vi "vis_acq_disassemble_finitePostproc.vi"(7 "error in":errorcluster) -> (20 "All Images Out":T1[](array[plugin-control]), 27 "error out":errorcluster)   [LabVIEW 2013]
doc: "Creates, and edits acquisitions using the NI Vision Acquisition Express VI.\n\nThe NI Vision Acquisition Wizard is launched by placing the Express VI on the block diagram. Select an acquisition source and configure an acquisition using NI-IMAQ, NI-IMAQdx, or simulate an acquisition by reading an AVI or image files from a folder. After an acquisition is configured, select controls and indicators to be able to programmatically set in LabVIEW. Double-click the Vision Acquisition Express VI to edit the acquisition.\n\nNote: Any images created by the Express VI need to be disposed after use. Use the IMAQ Dispose.vi to cleanup the images output by the Express VI when they are no longer needed."
uses:
  <vilib>/vision/driver/Vision Acquisition Express Utility VIs.llb/Vision Acquisition Path Convert (String).vi
  <vilib>/vision/driver/NI_Vision_Acquisition_Software.lvlib
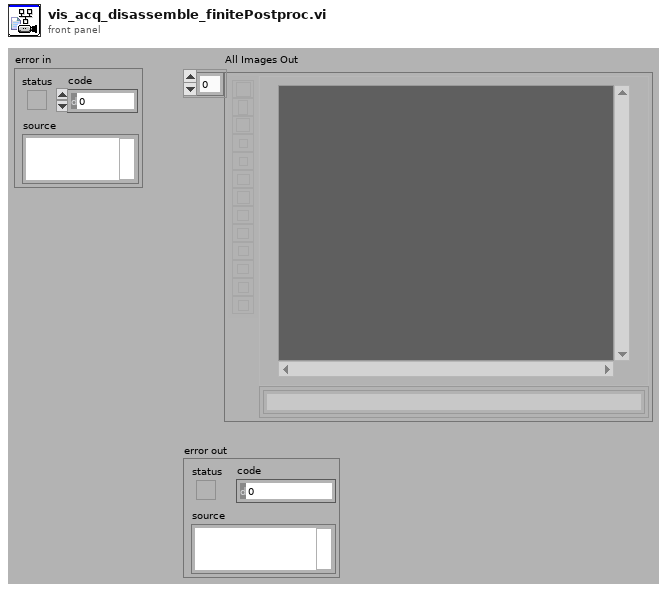
[diagram p1: front panel]
types:
  T1 = typedef "IMAQ Image.ctl" = refnum<image>
  T2 = typedef "IMAQdx.ctl" = refnum<k21>
  T3 = cluster{"File Type":string, "Quality":u32, "Compress":bool, "Lossless":bool, "Ratio":sgl, "Codec":string, "Frame Rate":u32, "Limit Frames":bool, "Max Frames":u32}
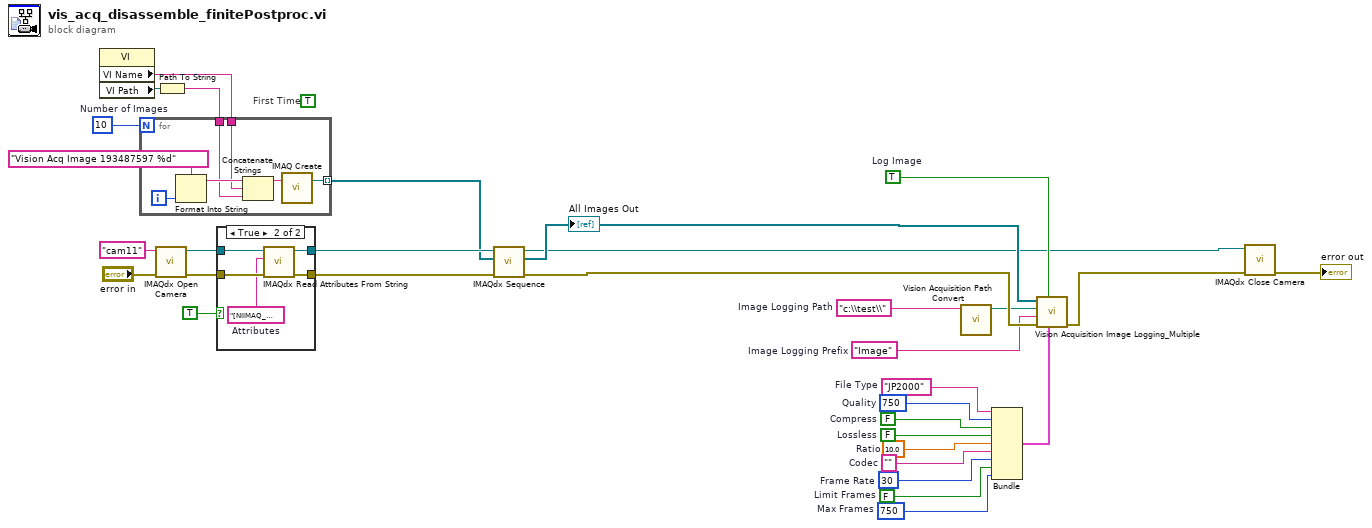
[diagram p0: block diagram]
diagram:
  w4 = "c:\\test\\"  # Image Logging Path
  w18 = "Image"  # Image Logging Prefix
  w6 = TRUE  # Log Image
  w12 = sgl 10.0  # Ratio
  w13 = FALSE  # Lossless
  w14 = FALSE  # Compress
  w15 = u32 750  # Quality
  w11 = ""  # Codec
  w10 = u32 30  # Frame Rate
  w8 = u32 750  # Max Frames
  w9 = FALSE  # Limit Frames
  w16 = "JP2000"  # File Type
  (unwired) TRUE
  w30 = u32 10  # Number of Images
  # "First Time"
  n1 = property class="VI"() -> ("VI Name"=w27:string, "VI Path"=w28:path)  [unwired: 2 in, 2 out]
  n2 = call <vilib>:"IMAQdx Open Camera.vi"("error in"="error in", "Session In"="cam11" ("Interface Name")) -> ("error out"=w24:errorcluster, "Session Out"=w25:T2)  [unwired: 1 in, 7 out]
  n3 = Path To String(path=w28) -> (string=w26:string)
  n4 = for {
    N: w30 -> [_]
    tunnel: [w38] -> w19 mode=indexing
    tunnel: w27 -> [w34]
    tunnel: w26 -> [w33]
    i -> [w37]
    n5 = Format Into String(format string="Vision Acq Image 193487597 %d" ("Image Name"), w37) -> (resulting string=w35:string)  [unwired: 2 in, 1 out]
    n6 = Concatenate Strings(w35, w34, w33) -> (w32:string)
    n7 = call "IMAQ Create"("Image Name"=w32) -> ("New Image"=w38:T1)  [unwired: 3 in, 2 out]
  }
  n8 = case shown="True" TRUE ("Init Attributes") {
    tunnel: w25 -> [w40 w45]
    tunnel: w24 -> [w39 w44]
    tunnel: [w40 w42] -> w20
    tunnel: [w39 w41] -> w23
    frame False {
    }
    frame True {
      w43 = "[NIIMAQ_HEADER]\nType = 2\nVersion = 8\n\n[CAMERA_DATA]\nAcquisitionAttributes::Bayer::Algorithm = \"Bilinear\"\nAcquisitionAttributes::Bayer::GainB = \"1\"\nAcquisitionAttributes::Bayer::GainG = \"1\"\nAcquisitionAttributes::Bayer::GainR = \"1\"\nAcquisitionAttributes::Bayer::Pattern = \"Use hardware value\"\nAcquisitionAttributes::BitsPerPixel = \"Use hardware value\"\nAcquisitionAttributes::IgnoreFirstFrame = \"false\"\nAcquisitionAttributes::ImageDecoderCopyMode = \"Auto\"\nAcquisitionAttributes::OutputImageType = \"Auto\"\nAcquisitionAttributes::OverwriteMode = \"Get Newest\"\nAcquisitionAttributes::PixelSignedness = \"Use hardware value\"\nAcquisitionAttributes::ReceiveTimestampMode = \"None\"\nAcquisitionAttributes::ShiftPixelBits = \"false\"\nAcquisitionAttributes::SwapPixelBytes = \"false\"\nAcquisitionAttributes::Timeout = \"5000\"\nAcquisitionAttributes::VerticalMirror = \"false\"\nAcquisitionAttributes::VideoMode = \"1280x720 RGB24 30.00fps\"\nCameraAttributes::BacklightCompensation::Mode = \"Manual\"\nCameraAttributes::BacklightCompensation::Value = \"false\"\nCameraAttributes::Brightness::Mode = \"Manual\"\nCameraAttributes::Brightness::Value = \"133\"\nCameraAttributes::Contrast::Mode = \"Manual\"\nCameraAttributes::Contrast::Value = \"0.050000000000000003\"\nCameraAttributes::Exposure::Mode = \"Auto\"\nCameraAttributes::Pan::Mode = \"Manual\"\nCameraAttributes::Pan::Value = \"0\"\nCameraAttributes::Saturation::Mode = \"Manual\"\nCameraAttributes::Saturation::Value = \"83\"\nCameraAttributes::Sharpness::Mode = \"Manual\"\nCameraAttributes::Sharpness::Value = \"25\"\nCameraAttributes::Tilt::Mode = \"Manual\"\nCameraAttributes::Tilt::Value = \"0\"\nCameraAttributes::WhiteBalance::Mode = \"Auto\"\nCameraAttributes::Zoom::Mode = \"Manual\"\nCameraAttributes::Zoom::Value = \"0\"\n"  # Attributes
      n9 = call <vilib>:"IMAQdx Read Attributes From String.vi"("error in"=w44, "Attributes String In"=w43, "Session In"=w45) -> ("error out"=w41:errorcluster, "Session Out"=w42:T2)  [unwired: 7 out]
    }
  }
  n10 = call <vilib>:"IMAQdx Sequence.vi"("error in"=w23, "Images In"=w19, "Session In"=w20) -> ("error out"=w21:errorcluster, "Images Out"=w5:T1[], "Session Out"=w1:T2)  [unwired: 6 out]
  "All Images Out" <- w5
  n11 = call-poly <vilib>:"Vision Acquisition Path Convert.vi"("Path In"=w4) -> ("Path Out"=w3:path)  [unwired: 10 in]
  n12 = Bundle("File Type"=w16, "Quality"=w15, "Compress"=w14, "Lossless"=w13, "Ratio"=w12, "Codec"=w11, "Frame Rate"=w10, "Limit Frames"=w9, "Max Frames"=w8) -> (w17:T3)  [unwired: 1 out]
  n13 = call <vilib>:"Vision Acquisition Image Logging_Multiple.vi"("File Settings"=w17, "Log Image"=w6, "error in (no error)"=w21, "Image Logging Prefix"=w18, "Image Logging Path"=w3, "All Images In"=w5) -> ("error out"=w7:errorcluster)  [unwired: 5 out]
  n14 = call <vilib>:"IMAQdx Close Camera.vi"("error in"=w7, "Session In"=w1) -> ("error out"=→"error out":errorcluster)  [unwired: 9 out]
